vi "Set Async Status.vi"(7 "State":T1, 8 "error in (no error)":errorcluster, 11 "Async Status in":refnum<queue>) -> (0 "error out":errorcluster, 3 "Async Status out":refnum<queue>)   [LabVIEW 2012, in "Waveform Data Logger Engine.lvlib"]
uses:
  Waveform Data Logger Engine.lvlib
  Types/Async Status.ctl
  Types/Async State.ctl
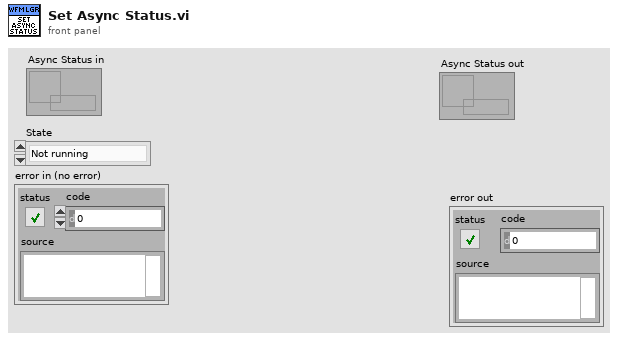
[diagram p1: front panel]
types:
  T1 = typedef "Waveform Data Logger Engine.lvlib/Async State.ctl" = enum16{"Not running", "Initializing", "Running", "Stopped"}
  T2 = typedef "Waveform Data Logger Engine.lvlib/Async Status.ctl" = cluster{"State":T1, "error":errorcluster}
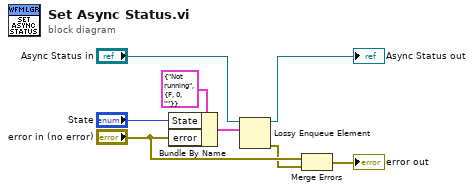
[diagram p0: block diagram]
diagram:
  n1 = Bundle By Name(cluster=T2 {"State"=enum."Not running", "error"={"status"=FALSE, "code"=0, "source"=""}} ("Async Status"), "State"="State", "error"="error in (no error)") -> (w6:T2)
  n2 = Lossy Enqueue Element(queue="Async Status in", element=w6) -> (queue out=→"Async Status out":refnum<queue>, error out=w2:errorcluster)  [unwired: 1 in, 2 out]
  n3 = Merge Errors("error in (no error)", w2) -> (→"error out":errorcluster)
